vi "rename libs.vi"(10 "User Project":refnum<vi>, 11 "NIVS_CDW_MetaDataObj in":refnum<class "NIVS_ScriptedModuleTemplate_MetaDataObj.lvclass">) -> (0 "error out":errorcluster)   [LabVIEW 2015, in "NIVS_ScriptedModuleTemplate_MetaDataObj.lvclass"]
uses:
  NIVS_ScriptedModuleTemplate_MetaDataObj.lvclass
  NIVS_ScriptedModuleTemplate_MetaDataObj.lvclass/NIVS_ScriptedModuleTemplate_MetaDataObj.ctl
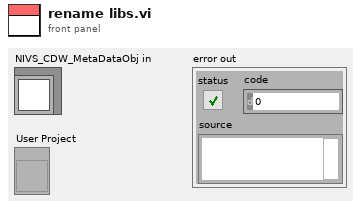
[diagram p1: front panel]
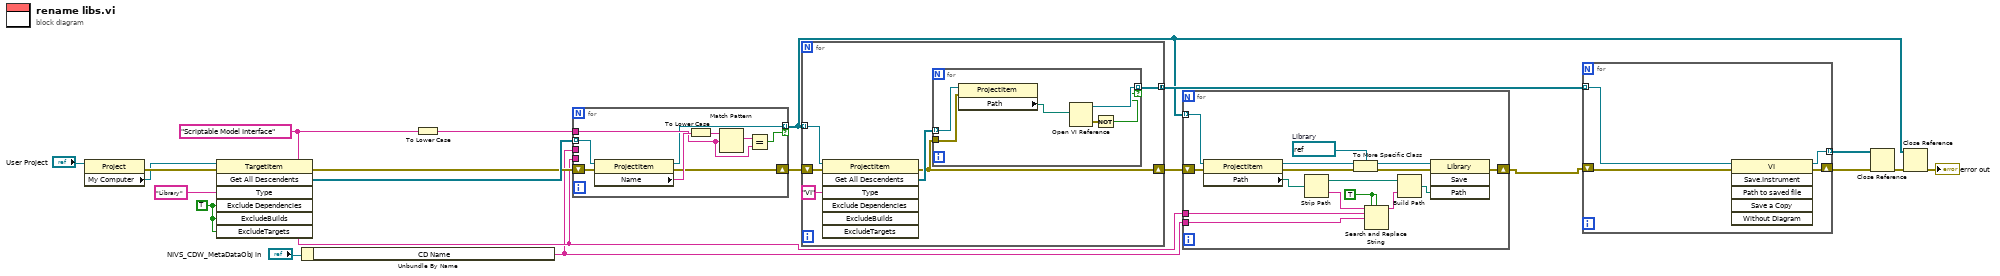
[diagram p0: block diagram]
diagram:
  w13 = TRUE ("ExcludeDependencies")
  w9 = "Scriptable Model Interface" ("Type")
  n1 = property class="Project"(reference="User Project") -> (error out=w17:errorcluster, "My Computer"=w15:refnum<vi>)  [unwired: 1 in, 1 out]
  n2 = invoke class="TargetItem" method="Get All Descendents"(reference=w15, error in=w17, "Type"="Library", "Exclude Dependencies"=w13, "ExcludeBuilds"=w13, "ExcludeTargets"=w13) -> (error out=w18:errorcluster, "All Descendents"=w19:refnum<vi>[])  [unwired: 1 in, 5 out]
  n3 = Unbundle By Name("NIVS_CDW_MetaDataObj in") -> ("CD Name"=w8:string)
  n4 = To Lower Case(string=w9) -> (all lower case string=w20:string)
  n5 = for {
    shift-right: [w23] -> w11
    shift-left: w18 -> [w29]
    tunnel: w19 -> [w28] mode=indexing
    tunnel: w20 -> [w24]
    tunnel: w9 -> [_]
    tunnel: w8 -> [_]
    tunnel: [w22] -> w3 mode=indexing if=w21
    n6 = property class="ProjectItem"(reference=w28, error in=w29) -> (reference out=w22:refnum<vi>, error out=w23:errorcluster, "Name"=w27:string)
    n7 = To Lower Case(string=w27) -> (all lower case string=w26:string)
    n8 = Match Pattern(string=w26, regular expression=w24) -> (match substring=w25:string)  [unwired: 1 in, 3 out]
    n9 = Equal?(x=w25, y=w24) -> (x = y?=w21:bool)
  }
  n10 = for {
    shift-right: [w32] -> w10
    shift-left: w11 -> [w35]
    tunnel: w3 -> [w34] mode=indexing
    tunnel: [w31] -> w7 mode=concatenating
    n11 = invoke class="ProjectItem" method="Get All Descendents"(reference=w34, error in=w35, "Type"="VI") -> (error out=w32:errorcluster, "All Descendents"=w33:refnum<vi>[])  [unwired: 4 in, 5 out]
    n12 = for {
      tunnel: w33 -> [w41] mode=indexing
      tunnel: w32 -> [w40]
      tunnel: [w38] -> w31 mode=indexing if=w36
      n13 = property class="ProjectItem"(reference=w41, error in=w40) -> ("Path"=w39:path)  [unwired: 2 out]
      n14 = Open VI Reference(vi path=w39) -> (vi reference=w38:refnum<vi>, error out=w37:errorcluster)  [unwired: 5 in]
      n15 = Not(x=w37) -> (.not. x?=w36:bool)
    }
  }
  n16 = for {
    shift-right: [w43] -> w2
    shift-left: w10 -> [w57]
    tunnel: w3 -> [w46] mode=indexing
    tunnel: w9 -> [w48]
    tunnel: w8 -> [w47]
    w49 = TRUE ("replace all? (F)")
    w50 = refnum<vi> refnum  # Library
    n17 = property class="ProjectItem"(reference=w46, error in=w57) -> (reference out=w51:refnum<vi>, error out=w56:errorcluster, "Path"=w55:path)
    n18 = Strip Path(path=w55) -> (stripped path=w53:path, name=w54:string)
    n19 = To More Specific Class(target class=w50, reference=w51, error in=w56) -> (specific class reference=w44:refnum<vi>, error out=w45:errorcluster)
    n20 = Search and Replace String(replace all?=w49, case sensitive?=w49, input string=w54, search string=w48, replace string=w47) -> (result string=w52:string)  [unwired: 3 in, 3 out]
    n21 = Build Path(base path=w53, name or relative path=w52) -> (appended path=w42:path)
    n22 = invoke class="Library" method="Save"(reference=w44, error in=w45, "Path"=w42) -> (error out=w43:errorcluster)  [unwired: 1 in, 3 out]
  }
  n23 = for {
    tunnel: w7 -> [w60] mode=indexing
    tunnel: [w61] -> w4 mode=indexing
    shift-right: [w58] -> w1
    shift-left: w2 -> [w59]
    n24 = invoke class="VI" method="Save.Instrument"(reference=w60, error in=w59) -> (reference out=w61:refnum<vi>, error out=w58:errorcluster)  [unwired: 4 in, 4 out]
  }
  n25 = Close Reference(reference=w4, error in (no error)=w1) -> (error out=w6:errorcluster)
  n26 = Close Reference(reference=w3, error in (no error)=w6) -> (error out=→"error out":errorcluster)
